vi "PXI4472與PXI6229 noise 測試.vi"() -> ()   [LabVIEW 2010]
uses:
  <vilib>/measure/maspectr.llb/FFT Spectrum (Mag-Phase) for 1 Chan.vi
  <vilib>/measure/NI_MAPro.lvlib
panel:
  out "Waveform Graph 2":waveform(dbl)(graph)
  out "Waveform Graph":cluster{"f0":dbl, "df":dbl, "magnitude":dbl[]}(graph)
  in  "stop (F)":bool
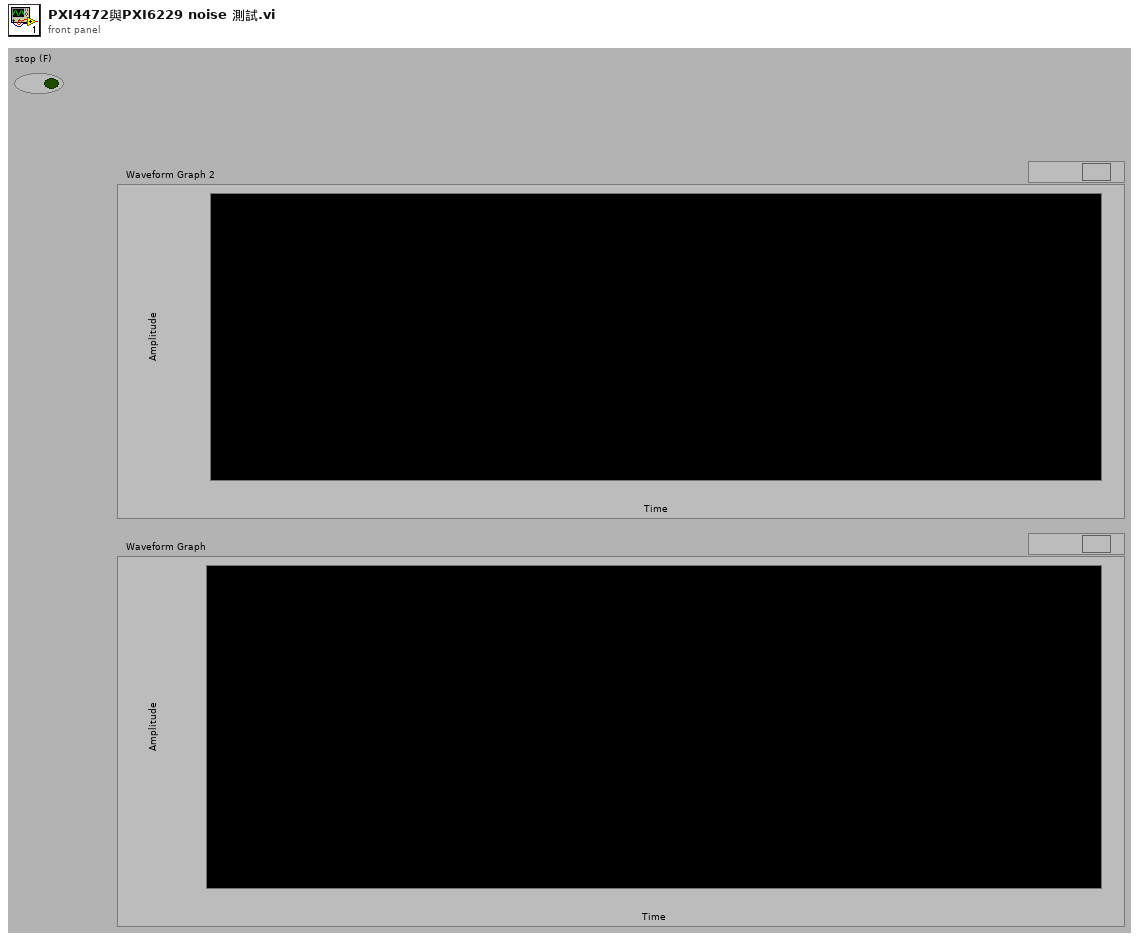
[diagram p1: front panel]
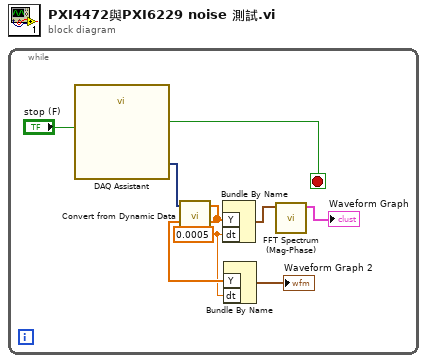
[diagram p0: block diagram]
diagram:
  n1 = while {
    stop <- w7 stop-if-true
    w2 = 0.0005 ("dt")
    n2 = call "DAQ Assistant"("stop (F)"="stop (F)") -> ("data"=w6:dynamicdata, "stopped"=w7:bool)  [unwired: 15 in, 2 out]
    n3 = call "Convert from Dynamic Data"("Dynamic Data Type"=w6) -> ("Array"=w3:dbl[])  [unwired: 3 in]
    n4 = Bundle By Name("Y"=w3, "dt"=w2) -> (w4:waveform(dbl))  [unwired: 1 in]
    n5 = Bundle By Name("Y"=w3, "dt"=w2) -> (→"Waveform Graph 2":waveform(dbl))  [unwired: 1 in]
    n6 = call-poly <vilib>:"FFT Spectrum (Mag-Phase).vi"("time signal"=w4) -> ("magnitude"=→"Waveform Graph":cluster{"f0":dbl, "df":dbl, "magnitude":dbl[]})  [unwired: 6 in, 4 out]
  }
